vi "Select Camera.vi"(4 "error in (no error)":errorcluster, 7 "camera":i32) -> (0 "error out":errorcluster, 3 "function return":i32)   [LabVIEW 2020, in "ThorConfocal.lvlib"]
doc: "long SelectCamera(const long camera);"
uses:
  ThorConfocal.lvlib
  ThorConfocal.dll
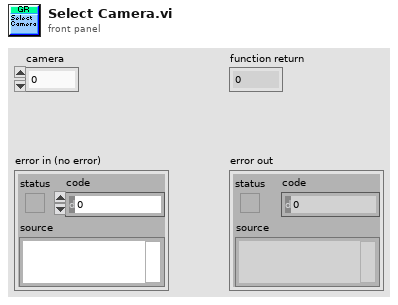
[diagram p1: front panel]
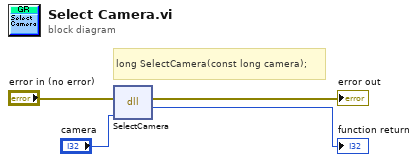
[diagram p0: block diagram]
diagram:
  # "long SelectCamera(const long camera);"
  n1 = dll-call lib="D:/software/TweezerTron Project/Instruments/Thorlabs/LSM_SDK/ThorConfocal.dll" fn="SelectCamera"(error in="error in (no error)", "camera"="camera") -> (error out=→"error out":errorcluster, "return type"=→"function return":i32)  [unwired: 3 in, 1 out]
